vi "FestoCPX.Station.Prod.Wait.vi"(8 "error in":errorcluster, 10 "Position":T2, 11 "Slot":T1) -> (0 "error out":errorcluster)   [LabVIEW 2015]
uses:
  Station/Station.ValvePosition.ctl
  Station/Station.ProductSlot.ctl
  tools/EventLog/EventLog.EventSource.ctl
  tools/Translator/Translator.Message.ctl
  Station/Station.ProductSuctionGripper.Type.ctl
  FestoCPX.DO.Signal.ctl
  FestoCPX.DI.Signal.ctl
  FestoCPX.Valve(1out1in).vi
  tools/EventLog/EventLog.CreateError(array).vi
  FestoCPX.DO.Data.Set.vi
  FestoCPX.DO.Data.State.Set.vi
  FestoCPX.DI.Data.State.Get.vi
  FestoCPX.DI.Data.States.Get.vi
  tools/User/User.Global.vi
  tools/EventLog/EventLog.New.vi
  tools/EventLog/EventLog.New(array).vi
  tools/ErrorHandling/ErrorHandling.Create.vi
panel:
  in  "Sucker (-1: Final)":i32=-1
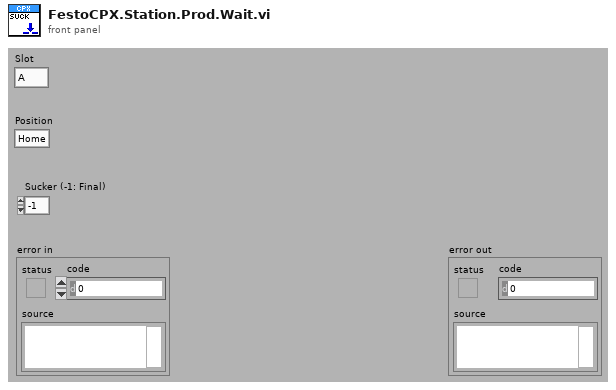
[diagram p1: front panel]
types:
  T1 = typedef "Station.ProductSlot.ctl" = enum8{"A", "B"}
  T2 = typedef "Station.ValvePosition.ctl" = enum16{"Home", "Work"}
  T3 = typedef "Station.ProductSuctionGripper.Type.ctl" = enum8{"Final A", "Final B", "Slot 1 A", "Slot 1 B", "Slot 2 A", "Slot 2 B", "Slot 3 A", "Slot 3 B", "Slot 4 A", "Slot 4 B"}
  T4 = typedef "Translator.Message.ctl" = enum16{"-", "Event confirmed", "Log out", "Log in", "Shutdown", "Cancel", "Start", "On", "Off", "OK", "NOK", "NOK %s", "Home", "Work", "Close", "Open", "In progress...", "Missing", "Empty", "Hardware failure", "Initial", "Error %d >> %s", "Error %d >> %s >> %s", "Msg %d >> %s", "Unable to reset Laser Interlock (%s)", "Unable to reset Laser Shutterlock. Laser not ready  (%s)", "Laser marking timeout", "Laser marking aborted", "Starting %s", "Quitting %s", "Configured", "Initializing", "Quitting", "Loading", "Running", "Stopped", "Summary", "Laser", "Do you want to continue?", "Press confirm button", "Station is not based. Do you want to exit?", "Station requires changeover. Do you want to run the test?", "Test options are not set as default. Do you want to continue?", "Product not detected. Do you want to continue?", "Product scan failed. Do you want to continue?", "Calibration", "Log out?", "System", "All", "IDLE", "Translating...%s", "Not found", "Alarm %s", "Run", "Skip", "Abort", "Repeat", "Please wait...", "Database disconnected", "Database disconnected - changeover disabled!", "Login to database successful", "Login to database failed: %d; %s", "Unable to check the product status of reference %d - database disconnected", "Unable to set the product status of reference %d - database disconnected", "Variant file backup %s", "Read steps (%s)", "Result", "Station armed!", "Station requires changeover!", "Select reference number...", "EMERGENCY BUTTON - press Control button", "EMERGENCY DOOR - press Control button", "Resetting Emergency...", "Unable to reset safety circuit - Emergency Button pressed", "Unable to reset safety circuit - Emergency Front Door open", "Unable to reset safety circuit - Emergency Side Door open", "Station not based", "Station not empty", "Station basing...", "Unkown reference", "Reference %d missing", "Reference invalid", "Wrong revolver", "Container missing", "Door open", "Close the front door", "Press start button", "Test done. Open the front door", "Test %s", "Test OK", "Test NOK", "Test error - press Confirm button", "Test stopped", "Remove product", "Confirm failure", "Test running...", "Test running... %.1f %%", "Stopping test...", "Finalizing test...", "Sequence folder '%s' is missing", "File '%s' is missing", "File '%s' is broken", "File '%s' is running", "Log file '%s' started", "Step '%s' added to log file", "Step '%s' graph added to log file", "Log file '%s' ended", "Log file '%s' ignored", "Log file '%s' exported", "Log file '%s' export failed", "Wrong serial number in log file", "Wrong reference number in log file", "Test steps are missing", "%s = %.3f", "Process param '%s' not found in DB", "Process param '%s' wrong order", "Process param '%s' value %.3f out of limits (%.3f; %.3f)", "Step%d param '%s' not found in DB", "Step%d param '%s' wrong order", "Step%d param '%s' value %.3f out of limits (%.3f; %.3f)", "Step%d EV '%s' not found in DB", "Step%d EV '%s' wrong order", "\"%s\" not found in DB", "\"%s\" wrong order", "\"%s\" value %.3f out of limits (%.3f; %.3f)", "\"%s\" not found in software", "Sequence initialized (%d)", "Sequence started", "Sequence done", "Sequence aborted", "Sequence aborted at work", "Sequence aborted at home", "Sequence error", "Seqeunce error at home", "Sequence error at work", "Unable to unload the slot %s. Product missing in the slot", "Unable to unload the slot %s. Product already in the arm", "Unable to accept the product as OK. Product missing in slot %s", "Unable to accept the product as OK. Product could not drop into the container at slot %s", "Unable to accept the product as NOK. Product could not drop into the container at slot %s", "Scan failed. Error %s", "Scan failed. Scanner disconnected", "Scan failed. Wrong Wabco number %d, limit (%d,%d)", "Scan failed. Wrong serial number %d, limit (%d,%d)", "Scan failed. Wrong date %d, limit (%d,%d)", "Scan failed. Wrong product wabco number %d (expected %d)", "Scan failed. Wrong product serial number %d (expected > 0)", "Scan OK %s", "%s = %d", "%s = %d->%d", "Unable to set %s = %.2f - Air Pressure Inside off", "Unable to reset Emergency Circuit - emg button", "Unable to reset Emergency Circuit - light curtain", "Unable to reset Emergency Circuit - door open", "Unable to set digital output '%s' = %d", "Unable to activate air pressure inside - timeout", "Unable to activate air pressure inside - aborted", "Unable to switch on Air Main Valve - Air Pressure Inlet off", "Unable to switch on Air Main Valve - Door open", "Unable to switch off Air Main Valve - timeout", "Unable to switch off Air Main Valve - aborted", "Unable to rotate Table - timeout", "Unable to rotate Table - aborted", "Unable to rotate Table - Air Pressure Inside off", "Unable to rotate Table - Product Lift A not in Home position", "Unable to rotate Table - Product Lift B not in Home position", "Unable to rotate Table - unlock before movement timeout", "Unable to rotate Table - lock after movement timeout", "Unable to move Table Lock to %s position - timeout", "Unable to move Table Lock to %s position - aborted", "Unable to move Table Lock to %s position - Air Pressure Inside off", "Unable to move Table Lock to %s position - Table not in position", "Unable to move Product Lift A to %s position - timeout", "Unable to move Product Lift B to %s position - timeout", "Unable to move Product Lift A to %s position - aborted", "Unable to move Product Lift B to %s position - aborted", "Unable to move Product Lift A to %s position - Air Pressure Inside off", "Unable to move Product Lift B to %s position - Air Pressure Inside off", "Unable to move Product Lift A to %s position - Table not locked", "Unable to move Product Lift B to %s position - Table not locked", "Unable to move Product Lift A to %s position - Product Arm not in Work position", "Unable to move Product Lift B to %s position - Product Arm not in Work position", "Unable to set Product Suction Gripper %s to %s - timeout", "Unable to set Product Suction Gripper %s to %s - aborted", "Unable to move Product Arm to %s position - timeout", "Unable to move Product Arm to %s position - aborted", "Unable to move Product Arm to %s position - Air Pressure Inside off", "Unable to move Product Arm to %s position - Product Lift A not in Home position", "Unable to move Product Arm to %s position - Product Lift B not in Home position", "Unable to move Product to %s position - timeout", "Unable to move Product to %s position - aborted", "Unable to move Product to %s position - Air Pressure Inside off", "Unable to move Product to %s position - Table not in position"}
  T5 = typedef "FestoCPX.DI.Signal.ctl" = enum16{"S.C. Emergency Stop", "S.C. Side Door Open", "S.C. Front Door Open", "Air Pressure Inlet", "Air Pressure Inside", "Door Close", "Button Start", "Button Stop", "Button Control", "Table Position", "Table Lock", "Product Arm OK", "Product Arm NOK", "Product Arm Work", "Product Lift A Home", "Product Lift B Home", "Product Move Home", "Product Move Work", "Revolver ID 1", "Revolver ID 2", "Revolver ID 3", "Revolver ID 4", "Revolver ID 5", "Product Slot 1 A Present", "Product Slot 1 B Present", "Product Slot 2 A Present", "Product Slot 2 B Present", "Product Slot 3 A Present", "Product Slot 3 B Present", "Product Slot 4 A Present", "Product Slot 4 B Present", "Product Final A Present", "Product Final B Present", "Product Output A Present", "Product Output B Present", "Product Container OK Present", "Product Container NOK Present"}
  T6 = typedef "FestoCPX.DO.Signal.ctl" = enum16{"Safety Reset", "Air Main Valve", "Door Lock", "Button LED Start", "Button LED Stop", "Button LED Control", "Traffic LED Red", "Traffic LED Orange", "Traffic LED Green", "Horn", "Laser Interlock", "Laser Shutterlock", "Laser Fume Extractor", "Product Suction Gripper Slot 1 A", "Product Suction Gripper Slot 1 B", "Product Suction Gripper Slot 2 A", "Product Suction Gripper Slot 2 B", "Product Suction Gripper Slot 3 A", "Product Suction Gripper Slot 3 B", "Product Suction Gripper Slot 4 A", "Product Suction Gripper Slot 4 B", "Product Suction Gripper Final A", "Product Suction Gripper Final B", "Q4 Table Turn Work", "Q4 Table Turn Home", "Q5 Product Lift A Home", "Q5 Product Lift B Home", "Q6 Product Move Work", "Q6 Product Move Home", "Q7 Product Arm OK", "Q7 Product Arm NOK", "Q8 Product Arm Work"}
  T7 = typedef "EventLog.EventSource.ctl" = enum16{"All", "Gui", "Ref", "File", "Seq", "Scan", "Lock", "AO", "AI", "CI", "DIO", "CPX", "PS", "Proda", "Trace", "Laser", "Scanner Prod", "Scanner Order"}
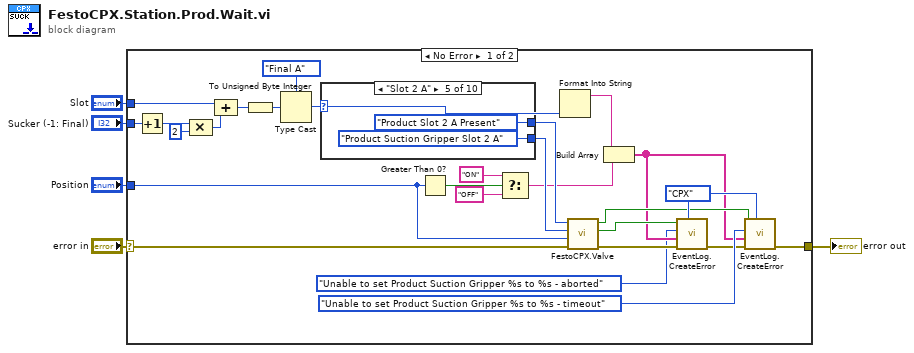
[diagram p0: block diagram]
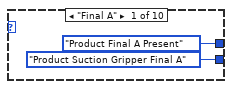
[diagram p2: hidden frame]
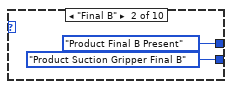
[diagram p3: hidden frame]
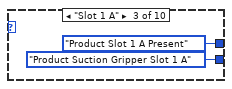
[diagram p4: hidden frame]
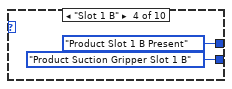
[diagram p5: hidden frame]
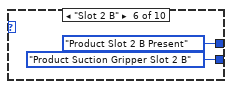
[diagram p6: hidden frame]
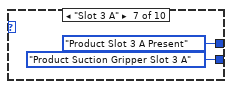
[diagram p7: hidden frame]
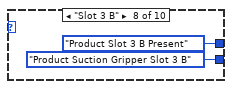
[diagram p8: hidden frame]
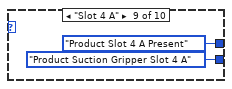
[diagram p9: hidden frame]
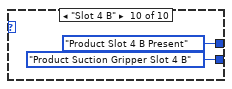
[diagram p10: hidden frame]
diagram:
  n1 = case shown="No Error" "error in" {
    selector: "error in" -> [w28 w53]
    tunnel: [w32 w53] -> w5
    tunnel: "Position" -> [w15 _]
    tunnel: "Sucker (-1: Final)" -> [w14 _]
    tunnel: "Slot" -> [w10 _]
    frame No Error {
      w22 = EventLog.EventSource."CPX" ("Source (All)")
      n2 = Increment(x=w14) -> (x+1=w8:i32)
      n3 = Compound Arithmetic op=MULTIPLY(w8, 2 ("value")) -> (w6:i32)
      n4 = Compound Arithmetic op=ADD(w10, w6) -> (w11:i32)
      n5 = To Unsigned Byte Integer(number=w11) -> (unsigned 8bit integer=w9:u8)
      n6 = Type Cast(type=Station.ProductSuctionGripper.Type."Final A" ("Type"), x=w9) -> (*(type *) &x=w13:T3)
      n7 = case shown="\"Slot 2 A\"" w13 {
        tunnel: [FestoCPX.DO.Signal."Product Suction Gripper Final A" ("CPX.DO") FestoCPX.DO.Signal."Product Suction Gripper Final B" ("CPX.DO") FestoCPX.DO.Signal."Product Suction Gripper Slot 1 A" ("CPX.DO") FestoCPX.DO.Signal."Product Suction Gripper Slot 1 B" ("CPX.DO") FestoCPX.DO.Signal."Product Suction Gripper Slot 2 A" ("CPX.DO") FestoCPX.DO.Signal."Product Suction Gripper Slot 2 B" ("CPX.DO") FestoCPX.DO.Signal."Product Suction Gripper Slot 3 A" ("CPX.DO") FestoCPX.DO.Signal."Product Suction Gripper Slot 3 B" ("CPX.DO") FestoCPX.DO.Signal."Product Suction Gripper Slot 4 A" ("CPX.DO") FestoCPX.DO.Signal."Product Suction Gripper Slot 4 B" ("CPX.DO")] -> w30
        tunnel: [FestoCPX.DI.Signal."Product Final A Present" ("DI") FestoCPX.DI.Signal."Product Final B Present" ("DI") FestoCPX.DI.Signal."Product Slot 1 A Present" ("DI") FestoCPX.DI.Signal."Product Slot 1 B Present" ("DI") FestoCPX.DI.Signal."Product Slot 2 A Present" ("DI") FestoCPX.DI.Signal."Product Slot 2 B Present" ("DI") FestoCPX.DI.Signal."Product Slot 3 A Present" ("DI") FestoCPX.DI.Signal."Product Slot 3 B Present" ("DI") FestoCPX.DI.Signal."Product Slot 4 A Present" ("DI") FestoCPX.DI.Signal."Product Slot 4 B Present" ("DI")] -> w29
        frame "Final A" {
        }
        frame "Final B" {
        }
        frame "Slot 1 A" {
        }
        frame "Slot 1 B" {
        }
        frame "Slot 2 A" {
        }
        frame "Slot 2 B" {
        }
        frame "Slot 3 A" {
        }
        frame "Slot 3 B" {
        }
        frame "Slot 4 A" {
        }
        frame "Slot 4 B" {
        }
      }
      n8 = Greater Than 0?(x=w15) -> (x > 0?=w16:bool)
      n9 = Select(t="ON" ("resulting string"), s=w16, f="OFF" ("resulting string")) -> (s? t:f=w24:string)
      n10 = Format Into String(w13) -> (resulting string=w27:string)  [unwired: 3 in, 1 out]
      n11 = call-poly "FestoCPX.Valve.vi"("error in (no error)"=w28, "Position"=w15, "Output"=w30, "Input"=w29) -> ("error out"=w19:errorcluster, "Aborted?"=w20:bool, "Timeout?"=w21:bool)  [unwired: 5 in]
      n12 = Build Array(w27, w24) -> (w18:string[])
      n13 = call-poly "EventLog.CreateError.vi"("Source (All)"=w22, "error in"=w19, "args"=w18, "msg"=Translator.Message."Unable to set Product Suction Gripper %s to %s - aborted", "create (T)"=w20) -> ("error out"=w23:errorcluster)  [unwired: 5 in, 1 out]
      n14 = call-poly "EventLog.CreateError.vi"("Source (All)"=w22, "error in"=w23, "args"=w18, "msg"=Translator.Message."Unable to set Product Suction Gripper %s to %s - timeout", "create (T)"=w21) -> ("error out"=w32:errorcluster)  [unwired: 5 in, 1 out]
    }
    frame Error {
    }
  }
  "error out" <- w5
